vi "Phonendoscope.vi"() -> ()   [LabVIEW 2016]
uses:
  <vilib>/Analysis/1siggen.llb/Ramp Pattern by Samples.vi
  <vilib>/express/express analysis/Spectral/Block/exnSpectralBlock spectral measurements power poly.vi
  <vilib>/express/express analysis/Spectral/Block/exnSpectralBlock spectral measurements power array WFM.vi
  <vilib>/addons/_NISVFA/_Baseband FFT/SVFA Power Spectrum (N Ch).vi
  <vilib>/express/express analysis/Spectral/Block/exnSpectralBlock spectral measurements power DDT.vi
  <vilib>/express/express analysis/Spectral/XNode/ExpressSpectralMeasurementsBlockNode.xnode
  <vilib>/Analysis/NI_AALPro.lvlib
  <vilib>/Analysis/NI_AAL_SigProc.lvlib
  <vilib>/Analysis/NI_AALBase.lvlib
panel:
  in  "Tab Control":T1(tab)
  out "Найдено":i32=4
  out "Время":dbl[](array[numeric])
  out "Амплитуда":dbl[](array[numeric])
  out "Входной сигнал":cluster{"Locations":dbl[], "Amplitudes":dbl[]}[](graph)
  in  "Порог":dbl(slide) scale=-2.0..2.0
  in  "Макс./Мин.":enum32{"Peaks", "Valleys"}(ring)
  out "AUDIO IN":bool
  out "FILE":bool
  in  "Перключение чтение с файла/myDAQ":bool
  in  "Чтение аудио файла":path
  in  "Запись аудио файла":path
  in  "ВКЛ/ВЫКЛ запись":bool
  out "Фильтр 3":bool
  out "Фильтр 2":bool
  in  "Выбор фильтра":i8(slide) scale=1.0..3.0
  out "Фильтр 1":bool
  out "Сигнал на звуковом выходе myDAQ \n(AUDIO OUT)":dynamicdata(graph)
  out "Преобразование Гильберта входного сигнала":dbl[](graph)
  out "Найдено":i32=4
  out "Время":dbl[](array[numeric])
  out "Амплитуда":dbl[](array[numeric])
  out "Сигнал на выходе фильтра 1":cluster{"Locations":dbl[], "Amplitudes":dbl[]}[](graph)
  in  "Порог":dbl(slide) scale=-2.0..2.0
  in  "Макс./Мин.":enum32{"Peaks", "Valleys"}(ring)
  out "Преобразование Гильберта сигнала на выходе фильтра 1":dbl[](graph)
  out "Найдено 2":i32=4
  out "Время 2":dbl[](array[numeric])
  out "Амплитуда 2":dbl[](array[numeric])
  out "Сигнал на выходе фильтра 2":cluster{"Locations":dbl[], "Amplitudes":dbl[]}[](graph)
  in  "Порог 2":dbl(slide) scale=-1.0..1.0
  in  "Макс./Мин. 2":enum32{"Peaks", "Valleys"}(ring)
  out "Преобразование Гильберта сигнала на выходе фильтра 2":dbl[](graph)
  out "Найдено 3":i32=4
  out "Время 3":dbl[](array[numeric])
  out "Амплитуда 3":dbl[](array[numeric])
  out "Сигнал на выходе фильтра 3":cluster{"Locations":dbl[], "Amplitudes":dbl[]}[](graph)
  in  "Порог 3":dbl(slide) scale=-1.5..1.5
  in  "Макс./Мин. 3":enum32{"Peaks", "Valleys"}(ring)
  out "Преобразование Гильберта сигнала на выходе фильтра 3":dbl[](graph)
  out "Спектральная мощность сигнала на входе":cluster{"f0":dbl, "df":dbl, "magnitude":dbl[]}[](graph)
  out "АЧХ на входе":cluster{"f0":dbl, "df":dbl, "magnitude":dbl[]}[](graph)
  out "Спектральная мощность сигнала на выходе фильтра 3":cluster{"f0":dbl, "df":dbl, "magnitude":dbl[]}[](graph)
  out "АЧХ на выходе фильтра 3":dynamicdata(graph)
  out "Спектральная мощность сигнала на выходе фильтра 2":cluster{"f0":dbl, "df":dbl, "magnitude":dbl[]}[](graph)
  out "АЧХ на выходе фильтра 2":dynamicdata(graph)
  out "Спектральная мощность сигнала на выходе фильтра 1":cluster{"f0":dbl, "df":dbl, "magnitude":dbl[]}[](graph)
  out "АЧХ на выходе фильтра 1":dynamicdata(graph)
  # "Виртуальная лаборатория LabVIEW для акустического анализа биомедицинских сигналов с электронного фонендоскопа"
  # "l"
  # "O"
  # "Управление звуковым выходом \nmyDAQ (AUDIO OUT)"
  # "Выбор фильтра"
  # "l"
  # "O"
  # "Фильтр Бесселя 7-ого порядка (20 Гц - 100 Гц)"
  # "Фильтр Бесселя 7-ого порядка (100 Гц - 300 Гц)"
  # "Фильтр Бесселя 7-ого порядка (20 Гц - 400 Гц)"
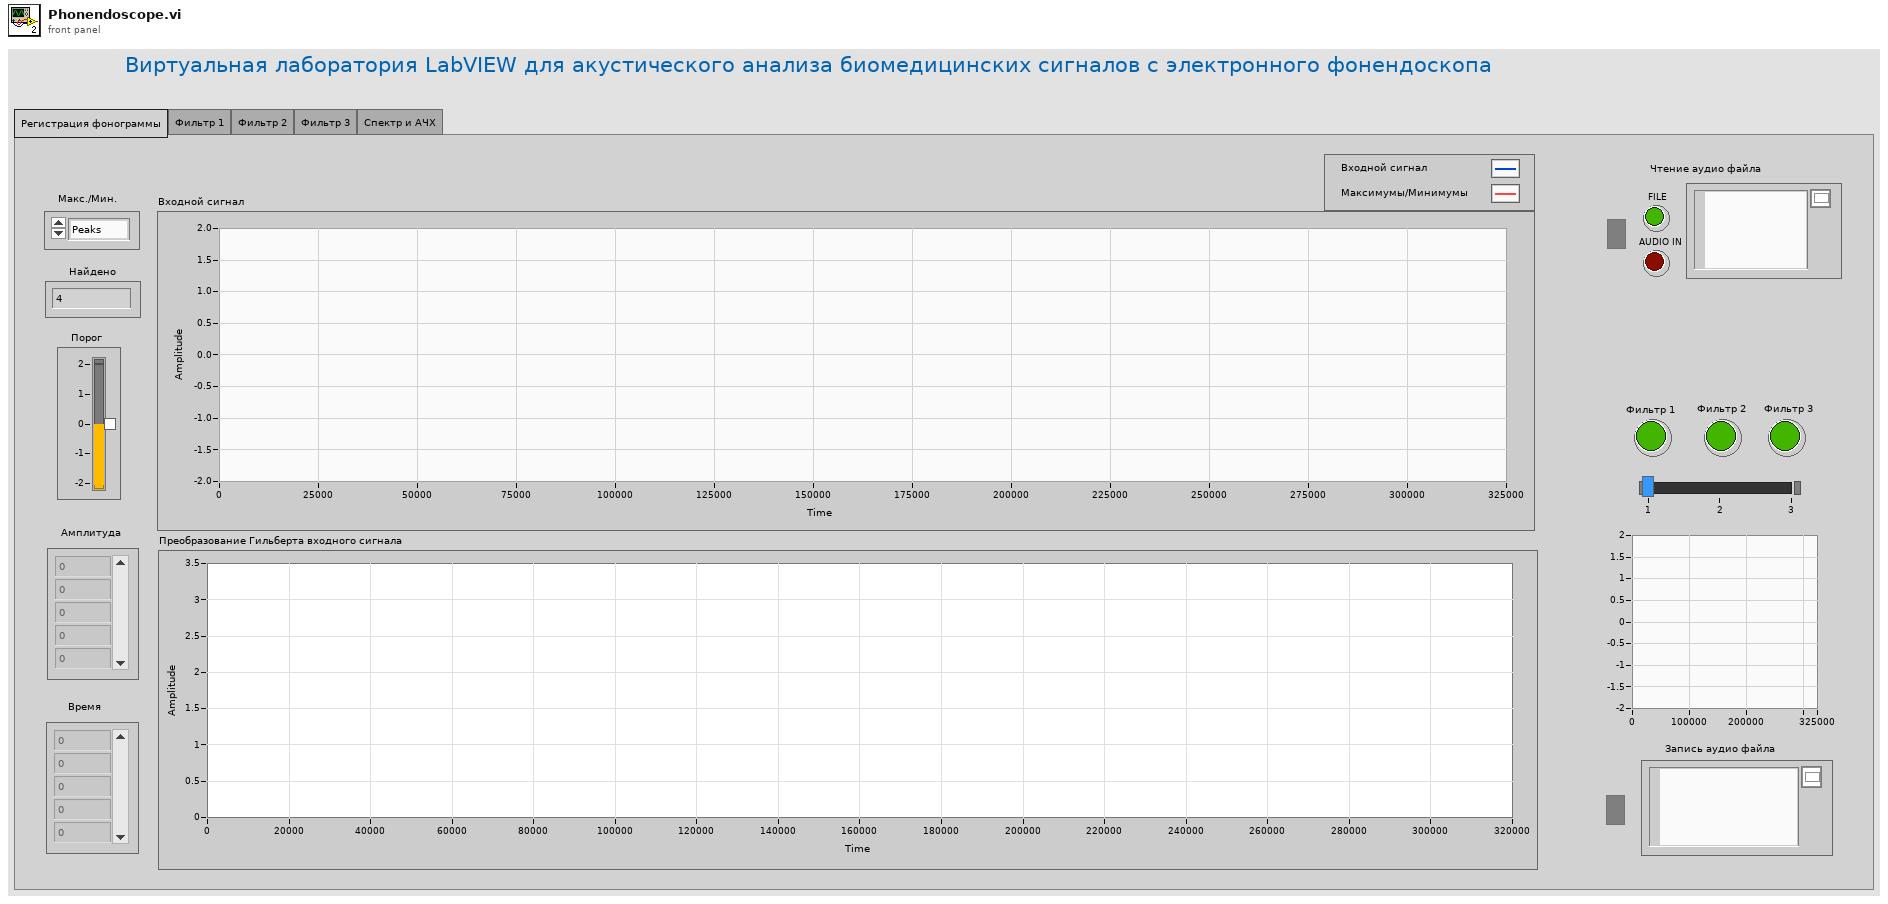
[diagram p1: front panel]
types:
  T1 = enum32{"Регистрация фонограммы", "Фильтр 1", "Фильтр 2", "Фильтр 3", "Спектр и АЧХ"}
  T2 = cluster{"averaging mode":u16, "weighting mode":u16, "number of averages":u32}
  T3 = cluster{"dB On (F)":bool, "unwrap phase (F)":bool, "convert to degree (F)":bool}
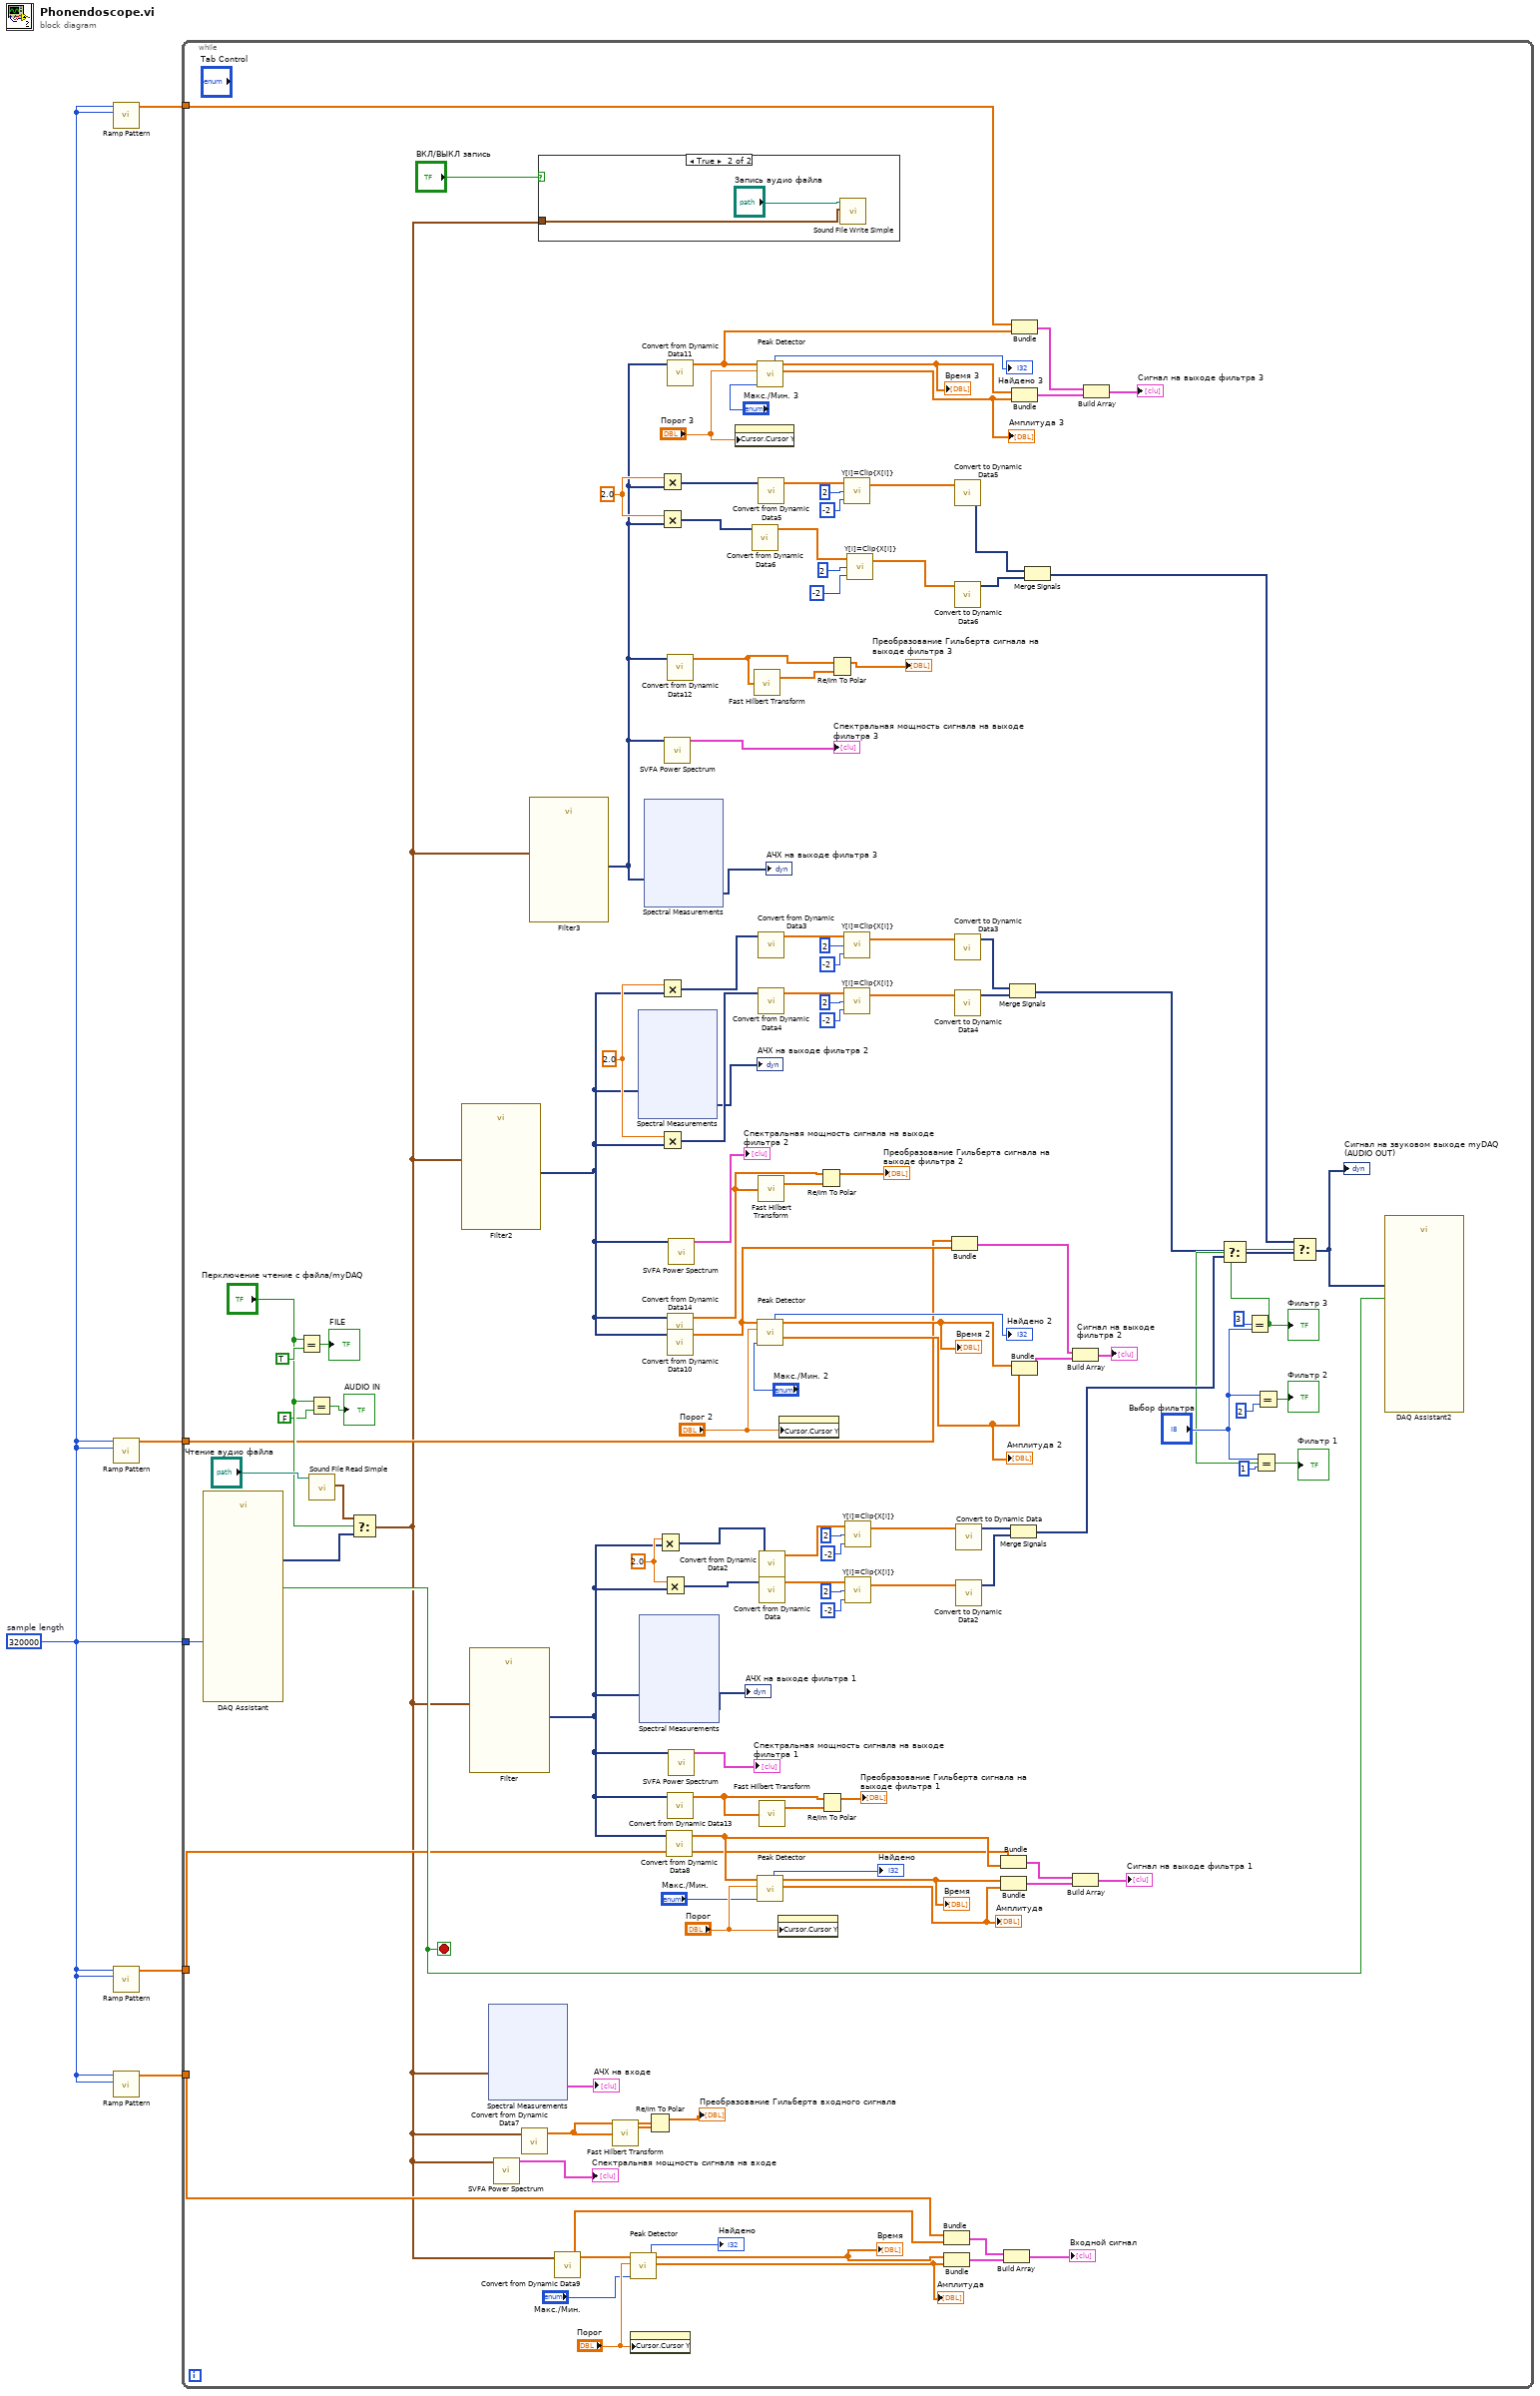
[diagram p0: block diagram]
diagram:
  w2 = 320000  # sample length
  n1 = call-poly <vilib>:"Ramp Pattern.vi"("end"=w2, "samples"=w2) -> ("Ramp Pattern"=w1:dbl[])  [unwired: 8 in, 1 out]
  n2 = call-poly <vilib>:"Ramp Pattern.vi"("end"=w2, "samples"=w2) -> ("Ramp Pattern"=w3:dbl[])  [unwired: 8 in, 1 out]
  n3 = call-poly <vilib>:"Ramp Pattern.vi"("end"=w2, "samples"=w2) -> ("Ramp Pattern"=w5:dbl[])  [unwired: 8 in, 1 out]
  n4 = call-poly <vilib>:"Ramp Pattern.vi"("end"=w2, "samples"=w2) -> ("Ramp Pattern"=w4:dbl[])  [unwired: 8 in, 1 out]
  n5 = while {
    tunnel: w2 -> [w61]
    tunnel: w5 -> [w60]
    tunnel: w4 -> [w50]
    tunnel: w3 -> [w39]
    tunnel: w1 -> [w29]
    stop <- w62 stop-if-true
    w100 = 2.0
    w117 = 2.0
    w130 = 2.0
    n6 = call "DAQ Assistant"("number of samples"=w61) -> ("data"=w78:dynamicdata, "stopped"=w62:bool)  [unwired: 15 in, 2 out]
    n7 = Equal?(x="Перключение чтение с файла/myDAQ", y=TRUE) -> (x = y?=→"FILE":bool)
    n8 = Equal?(x="Перключение чтение с файла/myDAQ", y=FALSE) -> (x = y?=→"AUDIO IN":bool)
    n9 = call <vilib>:"Sound File Read Simple.vi"("path"="Чтение аудио файла") -> ("data"=w77:waveform(dbl)[])  [unwired: 7 in, 3 out]
    n10 = Select(t=w77, s="Перключение чтение с файла/myDAQ", f=w78) -> (s? t:f=w14:waveform(dbl)[])
    n11 = call "Filter2"("Signal"=w14) -> ("Filtered Signal"=w6:dynamicdata)  [unwired: 9 in, 1 out]
    n12 = call "Filter"("Signal"=w14) -> ("Filtered Signal"=w18:dynamicdata)  [unwired: 9 in, 1 out]
    n13 = xnode "Spectral Measurements"("Signals"=w14) -> ("Power Spectrum"=→"АЧХ на входе":cluster{"f0":dbl, "df":dbl, "magnitude":dbl[]}[])  [unwired: 1 in, 1 out]
    n14 = call-poly <vilib>:"SVFA Power Spectrum.vi"("scaled signals [EU]"=w14) -> ("power spectra [dB EU]"=→"Спектральная мощность сигнала на входе":cluster{"f0":dbl, "df":dbl, "magnitude":dbl[]}[])  [unwired: 13 in, 5 out]
    n15 = call "Convert from Dynamic Data7"("Dynamic Data Type"=w14) -> ("Array"=w15:dbl[])  [unwired: 3 in]
    n16 = call "Filter3"("Signal"=w14) -> ("Filtered Signal"=w10:dynamicdata)  [unwired: 9 in, 1 out]
    n17 = case shown="True" "ВКЛ/ВЫКЛ запись" {
      tunnel: w14 -> [_ w132]
      frame False {
      }
      frame True {
        n18 = call <vilib>:"Sound File Write Simple.vi"("data"=w132, "path"="Запись аудио файла") -> ()  [unwired: 8 in, 2 out]
      }
    }
    n19 = call "Convert from Dynamic Data9"("Dynamic Data Type"=w14) -> ("Array"=w52:dbl[])  [unwired: 3 in]
    n20 = call <vilib>:"Fast Hilbert Transform.vi"("X"=w15) -> ("Hilbert{X}"=w16:dbl[])  [unwired: 1 out]
    n21 = call <vilib>:"Peak Detector.vi"("peaks/valleys"="Макс./Мин.", "threshold"="Порог", "X"=w52) -> ("Amplitudes"=w55:dbl[], "Locations"=w54:dbl[], "# found"=→"Найдено":i32)  [unwired: 4 in, 2 out]
    "Время" <- w54
    "Амплитуда" <- w55
    n22 = property on="Входной сигнал" class="XYGraph (strict)"("Cursor.Cursor Y"="Порог") -> ()  [unwired: 2 in, 2 out]
    n23 = xnode "Spectral Measurements"("Signals"=w6) -> ("Power Spectrum"=→"АЧХ на выходе фильтра 2":dynamicdata)  [unwired: 1 in, 1 out]
    n24 = xnode "Spectral Measurements"("Signals"=w18) -> ("Power Spectrum"=→"АЧХ на выходе фильтра 1":dynamicdata)  [unwired: 1 in, 1 out]
    n25 = xnode "Spectral Measurements"("Signals"=w10) -> ("Power Spectrum"=→"АЧХ на выходе фильтра 3":dynamicdata)  [unwired: 1 in, 1 out]
    n26 = Re/Im To Polar(2:w16, 3:w15) -> (1:→"Преобразование Гильберта входного сигнала":dbl[])  [unwired: 1 out]
    n27 = Multiply(x=w130, y=w18) -> (x*y=w127:dynamicdata)
    n28 = Multiply(x=w100, y=w10) -> (x*y=w97:dynamicdata)
    n29 = Multiply(x=w100, y=w10) -> (x*y=w91:dynamicdata)
    n30 = Multiply(x=w117, y=w6) -> (x*y=w114:dynamicdata)
    n31 = Multiply(x=w117, y=w6) -> (x*y=w108:dynamicdata)
    n32 = Multiply(x=w130, y=w18) -> (x*y=w121:dynamicdata)
    n33 = call-poly <vilib>:"SVFA Power Spectrum.vi"("scaled signals [EU]"=w10) -> ("power spectra [dB EU]"=→"Спектральная мощность сигнала на выходе фильтра 3":cluster{"f0":dbl, "df":dbl, "magnitude":dbl[]}[])  [unwired: 13 in, 5 out]
    n34 = call "Convert from Dynamic Data8"("Dynamic Data Type"=w18) -> ("Array"=w64:dbl[])  [unwired: 3 in]
    n35 = call "Convert from Dynamic Data11"("Dynamic Data Type"=w10) -> ("Array"=w31:dbl[])  [unwired: 3 in]
    n36 = call "Convert from Dynamic Data12"("Dynamic Data Type"=w10) -> ("Array"=w11:dbl[])  [unwired: 3 in]
    n37 = call "Convert from Dynamic Data14"("Dynamic Data Type"=w6) -> ("Array"=w7:dbl[])  [unwired: 3 in]
    n38 = call "Convert from Dynamic Data10"("Dynamic Data Type"=w6) -> ("Array"=w41:dbl[])  [unwired: 3 in]
    n39 = call "Convert from Dynamic Data13"("Dynamic Data Type"=w18) -> ("Array"=w20:dbl[])  [unwired: 3 in]
    n40 = call-poly <vilib>:"SVFA Power Spectrum.vi"("scaled signals [EU]"=w6) -> ("power spectra [dB EU]"=→"Спектральная мощность сигнала на выходе фильтра 2":cluster{"f0":dbl, "df":dbl, "magnitude":dbl[]}[])  [unwired: 13 in, 5 out]
    n41 = call-poly <vilib>:"SVFA Power Spectrum.vi"("scaled signals [EU]"=w18) -> ("power spectra [dB EU]"=→"Спектральная мощность сигнала на выходе фильтра 1":cluster{"f0":dbl, "df":dbl, "magnitude":dbl[]}[])  [unwired: 13 in, 5 out]
    n42 = property on="Сигнал на выходе фильтра 3" class="XYGraph (strict)"("Cursor.Cursor Y"="Порог 3") -> ()  [unwired: 2 in, 2 out]
    n43 = call "Convert from Dynamic Data6"("Dynamic Data Type"=w91) -> ("Array"=w90:dbl[])  [unwired: 3 in]
    n44 = call <vilib>:"Fast Hilbert Transform.vi"("X"=w11) -> ("Hilbert{X}"=w12:dbl[])  [unwired: 1 out]
    n45 = call <vilib>:"Peak Detector.vi"("peaks/valleys"="Макс./Мин.", "threshold"="Порог", "X"=w64) -> ("Amplitudes"=w67:dbl[], "Locations"=w66:dbl[], "# found"=→"Найдено":i32)  [unwired: 4 in, 2 out]
    "Время" <- w66
    "Амплитуда" <- w67
    n46 = call <vilib>:"Peak Detector.vi"("peaks/valleys"="Макс./Мин. 3", "threshold"="Порог 3", "X"=w31) -> ("Amplitudes"=w34:dbl[], "Locations"=w33:dbl[], "# found"=→"Найдено 3":i32)  [unwired: 4 in, 2 out]
    "Время 3" <- w33
    "Амплитуда 3" <- w34
    n47 = call <vilib>:"Peak Detector.vi"("peaks/valleys"="Макс./Мин. 2", "threshold"="Порог 2", "X"=w41) -> ("Amplitudes"=w44:dbl[], "Locations"=w43:dbl[], "# found"=→"Найдено 2":i32)  [unwired: 4 in, 2 out]
    "Время 2" <- w43
    "Амплитуда 2" <- w44
    n48 = call "Convert from Dynamic Data5"("Dynamic Data Type"=w97) -> ("Array"=w96:dbl[])  [unwired: 3 in]
    n49 = call "Convert from Dynamic Data3"("Dynamic Data Type"=w114) -> ("Array"=w113:dbl[])  [unwired: 3 in]
    n50 = call "Convert from Dynamic Data4"("Dynamic Data Type"=w108) -> ("Array"=w107:dbl[])  [unwired: 3 in]
    n51 = call <vilib>:"Fast Hilbert Transform.vi"("X"=w7) -> ("Hilbert{X}"=w8:dbl[])  [unwired: 1 out]
    n52 = call "Convert from Dynamic Data2"("Dynamic Data Type"=w127) -> ("Array"=w126:dbl[])  [unwired: 3 in]
    n53 = call "Convert from Dynamic Data"("Dynamic Data Type"=w121) -> ("Array"=w120:dbl[])  [unwired: 3 in]
    n54 = call <vilib>:"Fast Hilbert Transform.vi"("X"=w20) -> ("Hilbert{X}"=w21:dbl[])  [unwired: 1 out]
    n55 = property on="Сигнал на выходе фильтра 1" class="XYGraph (strict)"("Cursor.Cursor Y"="Порог") -> ()  [unwired: 2 in, 2 out]
    n56 = property on="Сигнал на выходе фильтра 2" class="XYGraph (strict)"("Cursor.Cursor Y"="Порог 2") -> ()  [unwired: 2 in, 2 out]
    n57 = Re/Im To Polar(2:w8, 3:w7) -> (1:→"Преобразование Гильберта сигнала на выходе фильтра 2":dbl[])  [unwired: 1 out]
    n58 = Re/Im To Polar(2:w21, 3:w20) -> (1:→"Преобразование Гильберта сигнала на выходе фильтра 1":dbl[])  [unwired: 1 out]
    n59 = Re/Im To Polar(2:w12, 3:w11) -> (1:→"Преобразование Гильберта сигнала на выходе фильтра 3":dbl[])  [unwired: 1 out]
    n60 = call <vilib>:"Y[i]=Clip{X[i]}.vi"("lower limit"=-2, "upper limit"=2, "Input Array"=w96) -> ("Clipped Array"=w95:dbl[])  [unwired: 1 out]
    n61 = call <vilib>:"Y[i]=Clip{X[i]}.vi"("lower limit"=-2, "upper limit"=2, "Input Array"=w113) -> ("Clipped Array"=w112:dbl[])  [unwired: 1 out]
    n62 = call <vilib>:"Y[i]=Clip{X[i]}.vi"("lower limit"=-2, "upper limit"=2, "Input Array"=w107) -> ("Clipped Array"=w106:dbl[])  [unwired: 1 out]
    n63 = call <vilib>:"Y[i]=Clip{X[i]}.vi"("lower limit"=-2, "upper limit"=2, "Input Array"=w126) -> ("Clipped Array"=w125:dbl[])  [unwired: 1 out]
    n64 = call <vilib>:"Y[i]=Clip{X[i]}.vi"("lower limit"=-2, "upper limit"=2, "Input Array"=w120) -> ("Clipped Array"=w119:dbl[])  [unwired: 1 out]
    n65 = call <vilib>:"Y[i]=Clip{X[i]}.vi"("lower limit"=-2, "upper limit"=2, "Input Array"=w90) -> ("Clipped Array"=w89:dbl[])  [unwired: 1 out]
    n66 = Bundle("Ramp Pattern"=w50, "Array"=w52) -> (w59:cluster{"Ramp Pattern":dbl[], "Array":dbl[]})  [unwired: 1 out]
    n67 = Bundle("Locations"=w54, "Amplitudes"=w55) -> (w57:cluster{"Locations":dbl[], "Amplitudes":dbl[]})  [unwired: 1 out]
    n68 = Bundle("Ramp Pattern"=w39, "Array"=w41) -> (w48:cluster{"Ramp Pattern":dbl[], "Array":dbl[]})  [unwired: 1 out]
    n69 = call "Convert to Dynamic Data5"("Array"=w95) -> ("Dynamic Data Type"=w94:dynamicdata)  [unwired: 3 in]
    n70 = call "Convert to Dynamic Data6"("Array"=w89) -> ("Dynamic Data Type"=w88:dynamicdata)  [unwired: 3 in]
    n71 = call "Convert to Dynamic Data3"("Array"=w112) -> ("Dynamic Data Type"=w111:dynamicdata)  [unwired: 3 in]
    n72 = call "Convert to Dynamic Data4"("Array"=w106) -> ("Dynamic Data Type"=w105:dynamicdata)  [unwired: 3 in]
    n73 = call "Convert to Dynamic Data"("Array"=w125) -> ("Dynamic Data Type"=w124:dynamicdata)  [unwired: 3 in]
    n74 = call "Convert to Dynamic Data2"("Array"=w119) -> ("Dynamic Data Type"=w118:dynamicdata)  [unwired: 3 in]
    n75 = Bundle("Ramp Pattern"=w60, "Array"=w64) -> (w71:cluster{"Ramp Pattern":dbl[], "Array":dbl[]})  [unwired: 1 out]
    n76 = Bundle("Locations"=w66, "Amplitudes"=w67) -> (w69:cluster{"Locations":dbl[], "Amplitudes":dbl[]})  [unwired: 1 out]
    n77 = Build Array(w59, w57) -> (→"Входной сигнал":cluster{"Locations":dbl[], "Amplitudes":dbl[]}[])
    n78 = Merge Signals(w111, w105) -> (w84:dynamicdata)
    n79 = Merge Signals(w124, w118) -> (w86:dynamicdata)
    n80 = Bundle("Ramp Pattern"=w29, "Array"=w31) -> (w38:cluster{"Ramp Pattern":dbl[], "Array":dbl[]})  [unwired: 1 out]
    n81 = Bundle("Locations"=w33, "Amplitudes"=w34) -> (w36:cluster{"Locations":dbl[], "Amplitudes":dbl[]})  [unwired: 1 out]
    n82 = Bundle("Locations"=w43, "Amplitudes"=w44) -> (w46:cluster{"Locations":dbl[], "Amplitudes":dbl[]})  [unwired: 1 out]
    n83 = Merge Signals(w94, w88) -> (w81:dynamicdata)
    n84 = Build Array(w48, w46) -> (→"Сигнал на выходе фильтра 2":cluster{"Locations":dbl[], "Amplitudes":dbl[]}[])
    n85 = Build Array(w71, w69) -> (→"Сигнал на выходе фильтра 1":cluster{"Locations":dbl[], "Amplitudes":dbl[]}[])
    n86 = Build Array(w38, w36) -> (→"Сигнал на выходе фильтра 3":cluster{"Locations":dbl[], "Amplitudes":dbl[]}[])
    n87 = Equal?(x="Выбор фильтра", y=i8 3) -> (x = y?=w83:bool)
    "Фильтр 3" <- w83
    n88 = Equal?(x="Выбор фильтра", y=i8 1) -> (x = y?=w85:bool)
    "Фильтр 1" <- w85
    n89 = Select(t=w86, s=w85, f=w84) -> (s? t:f=w82:dynamicdata)
    n90 = Equal?(x="Выбор фильтра", y=i8 2) -> (x = y?=→"Фильтр 2":bool)
    n91 = Select(t=w81, s=w83, f=w82) -> (s? t:f=w49:dynamicdata)
    "Сигнал на звуковом выходе myDAQ \n(AUDIO OUT)" <- w49
    n92 = call "DAQ Assistant2"("data"=w49, "stop (F)"=w62) -> ()  [unwired: 15 in, 3 out]
  }
